vi "UI.vi"(8 "error in (no error)":errorcluster, 11 "Add in":refnum<class "Add.lvclass">) -> (0 "error out":errorcluster, 3 "Add out":refnum<class "Add.lvclass">)   [LabVIEW 2020, in "Add.lvclass"]
uses:
  Add.lvclass
  C:/Users/khishore.kumar/Khishore/labview_tips_2024/src/Assignment 25/Arithmetic Operations/Arithmetic Operations.lvclass
  Arithmetic Operations.lvclass/Arithmetic Operations.ctl
  Accessors/Write/Write A.vi
  Accessors/Write/Write B.vi
  Accessors/Read/Read C.vi
panel:
  out "C":dbl
  in  "B":dbl
  in  "A":dbl
  # "ADD"
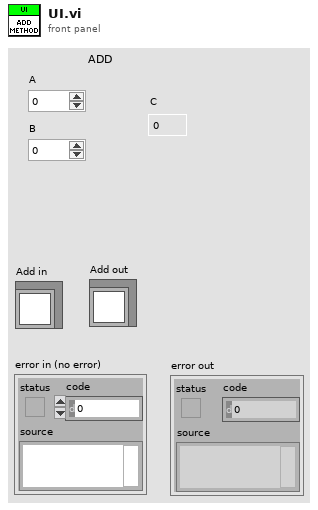
[diagram p1: front panel]
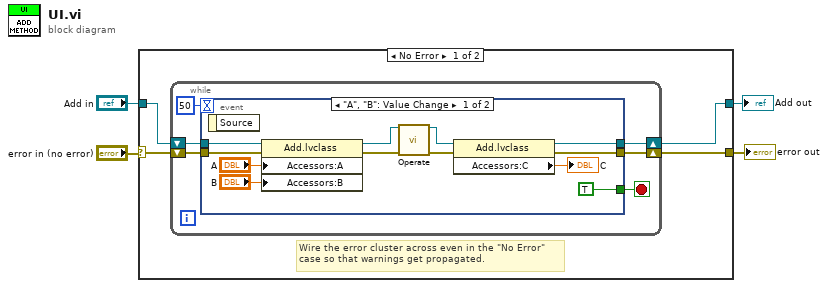
[diagram p0: block diagram]
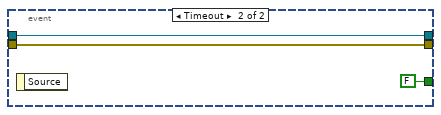
[diagram p2: hidden frame]
diagram:
  n1 = case shown="No Error" "error in (no error)" {
    selector: "error in (no error)" -> [w8 w31]
    tunnel: [w6 w31] -> w3
    tunnel: [w5 w30] -> w1
    tunnel: "Add in" -> [w7 w30]
    frame No Error {
      # "Wire the error cluster across even in the \"No Error\"\ncase so that warnings get propagated."
      n2 = while {
        shift-right: [w12] -> w6
        shift-left: w8 -> [w14]
        shift-right: [w11] -> w5
        shift-left: w7 -> [w13]
        stop <- w9 stop-if-true
        n3 = event shown="[0] \"A\", \"B\": Value Change" {
          selector: _ -> [_ _]
          dyn-events: _ -> [_ _]
          timeout: 50 -> [_ _]
          tunnel: w14 -> [w26 w28]
          tunnel: w13 -> [w25 w29]
          tunnel: [w17 w28] -> w12
          tunnel: [w16 w29] -> w11
          tunnel: [TRUE FALSE] -> w9
          event "A", "B": Value Change {
            n4 = event-data() -> ()  [unwired: 1 in, 1 out]
            n5 = property class="Add.lvclass"(reference=w25, error in=w26, "Accessors:A"="A", "Accessors:B"="B") -> (reference out=w21:refnum<class "Add.lvclass">, error out=w22:errorcluster)
            n6 = call-dynamic "Operate.vi"("Add in"=w21, "error in (no error)"=w22) -> ("Add out"=w20:refnum<class "Add.lvclass">, "error out"=w19:errorcluster)  [unwired: 12 in]
            n7 = property class="Add.lvclass"(reference=w20, error in=w19) -> (reference out=w16:refnum<class "Add.lvclass">, error out=w17:errorcluster, "Accessors:C"=→"C":dbl)
          }
          event Timeout {
            n8 = event-data() -> ()  [unwired: 1 in, 1 out]
          }
        }
      }
    }
    frame Error {
    }
  }
  "error out" <- w3
  "Add out" <- w1
